vi "ADIS16460_Loop.vi"(8 "error in":errorcluster, 11 "ADI IMU Interrupt DevRef":T1={"ADI IMU DevRef"={"DevStatus"={"status"=FALSE, "code"=0, "source"=""}, "Handle"=0, "SPI Bus"=enum."SPI On-Board, CS0", "Device Found"=FALSE, "Device Ready"=FALSE, "Yaw Axis"=enum."Z", "AHRS Algorithm"=enum."Complementary"}, "InterruptRef"={"DevStatus"={"status"=FALSE, "code"=0, "source"=""}, "InterruptIndex"=enum."0"}}) -> (0 "error out":errorcluster, 1 "Device Found":bool)   [LabVIEW 2015, in "FRC ADIS16460.lvlib"]
doc: "Periodically reads the ADI MXP IMU valuse and makes data available for use elsewhere in your robot project. Place this block within PeriodicTasks.vi outside any loops."
uses:
  FRC ADIS16460.lvlib
  WPI_ADIS16460_InterruptDevRef.ctl
  WPI_ADIS16460_DevRef.ctl
  <vilib>/Rock Robotics/SystemInterfaces/spilib/spi_bus.ctl
  <vilib>/Rock Robotics/WPI/Interrupt/WPI_InterruptRef.ctl
  <vilib>/Rock Robotics/SystemInterfaces/Interrupt/FPGA_InterruptIndex.ctl
  <vilib>/Rock Robotics/WPI/SPI/WPI_SPIDevRef.ctl
  <vilib>/Platform/TimedLoop/XDataNode/timing_clust.ctl
  <vilib>/Platform/TimedLoop/XDataNode/nitl_modes.ctl
  <vilib>/Platform/TimedLoop/XDataNode/wakeup.ctl
  <vilib>/Analysis/baseanly.llb/Mean (DBL).vi
  <vilib>/Rock Robotics/SystemInterfaces/Interrupt/FPGA_WaitOnInterrupt.vi
  <vilib>/Rock Robotics/WPI/Utilities/WPI_UtilitiesTimebaseConstants.vi
  <vilib>/Rock Robotics/SystemInterfaces/Interrupt/FPGA_InterruptReadTimestamp.vi
  <vilib>/platform/TimedLoop/XDataNode/XDataNode.xnode
  <vilib>/Platform/TimedLoop/XDataNode/XDNodeRunTimeDep.lvlib
  <vilib>/Analysis/NI_AALBase.lvlib
panel:
  out "Loop Verification":i32
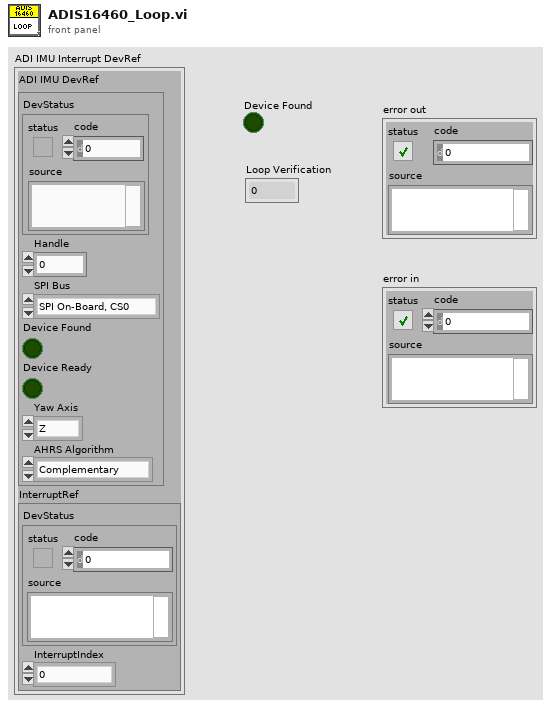
[diagram p1: front panel]
types:
  T1 = typedef "FRC ADIS16460.lvlib/WPI_ADIS16460_InterruptDevRef.ctl" = cluster{"ADI IMU DevRef":T2, "InterruptRef":T4}
  T2 = typedef "FRC ADIS16460.lvlib/WPI_ADIS16460_DevRef.ctl" = cluster{"DevStatus":errorcluster, "Handle":i32, "SPI Bus":T3, "Device Found":bool, "Device Ready":bool, "Yaw Axis":enum16{"X", "Y", "Z"}, "AHRS Algorithm":enum16{"Complementary", "Madgwick"}}
  T3 = typedef "spi_bus.ctl" = enum16{"SPI On-Board, CS0", "SPI On-Board, CS1", "SPI On-Board, CS2", "SPI On-Board, CS3", "SPI MXP", "Invalid"}
  T4 = typedef "WPI_InterruptRef.ctl" = cluster{"DevStatus":errorcluster, "InterruptIndex":T5}
  T5 = typedef "FPGA_InterruptIndex.ctl" = enum8{"0", "1", "2", "3", "4", "5", "6", "7", "Invalid"}
  T6 = typedef "WPI_SPIDevRef.ctl" = cluster{"DevStatus":errorcluster, "Handle":i32, "SPI Bus":T3}
  T7 = typedef "XDNodeRunTimeDep.lvlib/timing_clust.ctl" = cluster{"Expected End [f-1]":u64, "Actual End [f-1]":u64, "Finished Late? [f-1]":bool, "Expected End [i-1]":u64, "Actual End [i-1]":u64, "Finished Late? [i-1]":bool, "Expected Start [i]":u64, "Actual Start [i]":u64, "Expected Start [f]":u64, "Actual Start [f]":u64, "Source Name":string, "Structure Name":string, "Period":i64, "Deadline":i64, "Offset":i64, "Start":i64, "Priority":i32, "Timeout":i32, "Mode":T8, "Wakeup Reason":T9, "Error":errorcluster, "Source Type":string, "Secondary Source Type":string, "Global End Time":u64, "Global Start Time":u64, "Frame Duration":u64, "Iteration Duration":u64, "Assigned CPU":i32, "I/O Scan Engine Mode":u32}
  T8 = typedef "XDNodeRunTimeDep.lvlib/nitl_modes.ctl" = enum32{"No Change", "Process missed periods, maintain original phase", "Discard missed periods, maintain original phase", "Process missed periods, ignore original phase", "Discard missed periods, ignore original phase"}
  T9 = typedef "XDNodeRunTimeDep.lvlib/wakeup.ctl" = enum32{"Normal", "Aborted", "Asynchronous wakeup", "Timing source error", "Timed loop error", "Timeout"}
  T10 = cluster{"X Gyro Rate":dbl, "Y Gyro Rate":dbl, "Z Gyro Rate":dbl, "X Accel":dbl, "Y Accel":dbl, "Z Accel":dbl, "Temperature":dbl}
  T11 = cluster{"Output[0]":dbl, "Output[1]":dbl, "Output[2]":dbl}
  T12 = cluster{"Data Array[0]":dbl, "Data Array[1]":dbl, "Data Array[2]":dbl, "Data Array[3]":dbl, "Data Array[4]":dbl, "Data Array[5]":dbl, "Data Array[6]":dbl, "Data Array[7]":dbl, "Data Array[8]":dbl, "Data Array[9]":dbl, "Data Array[10]":dbl}
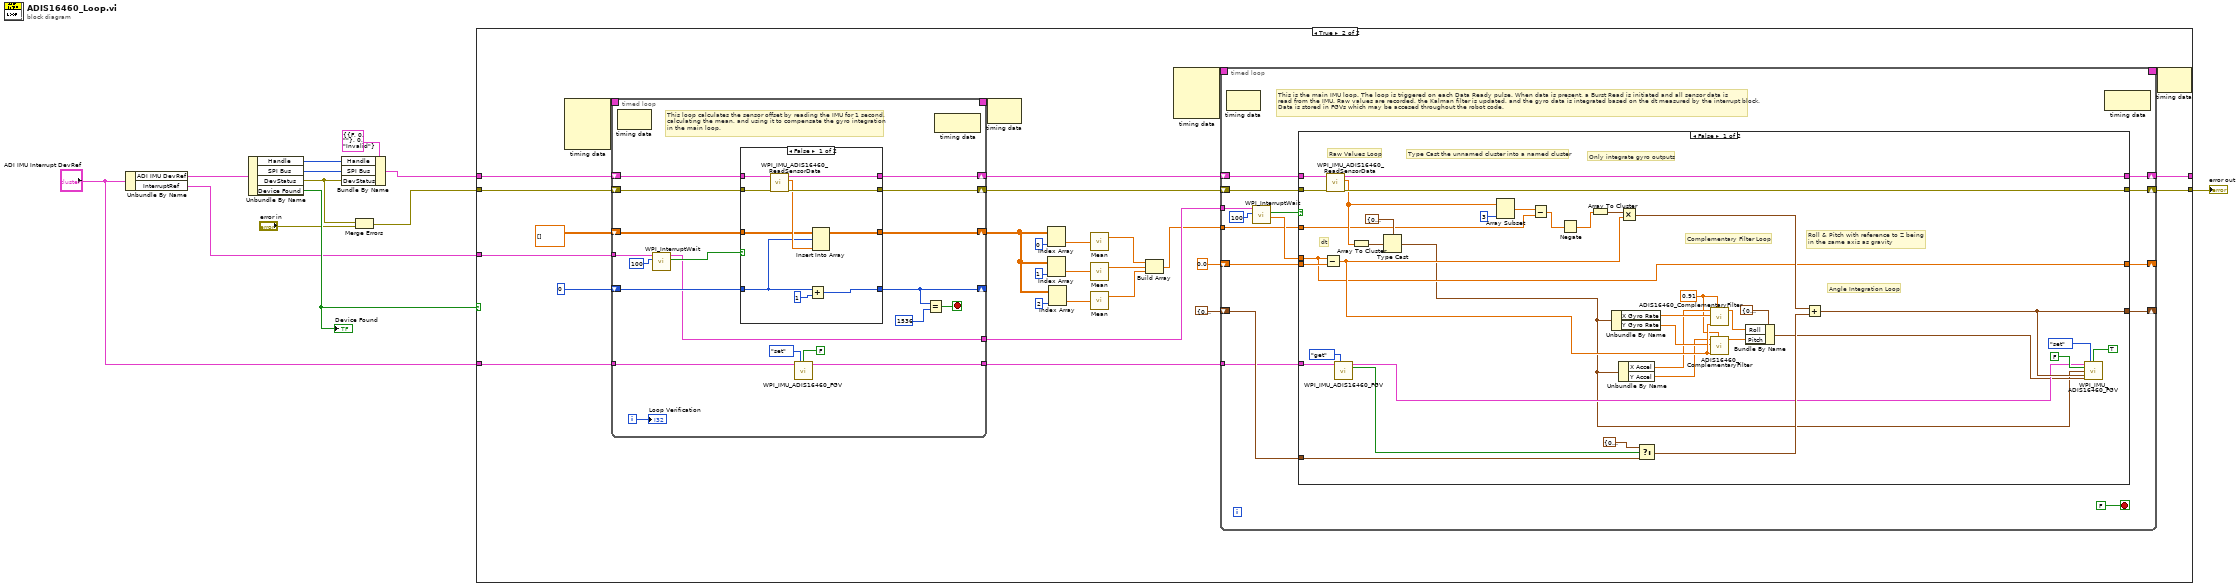
[diagram p0: block diagram]
diagram:
  n1 = Unbundle By Name("ADI IMU Interrupt DevRef") -> ("ADI IMU DevRef"=w6:T2, "InterruptRef"=w5:T4)
  n2 = Unbundle By Name(w6) -> ("Handle"=w11:i32, "SPI Bus"=w10:T3, "DevStatus"=w4:errorcluster, "Device Found"=w9:bool)
  "Device Found" <- w9
  n3 = Bundle By Name(cluster=T6 {"DevStatus"={"status"=FALSE, "code"=0, "source"=""}, "Handle"=0, "SPI Bus"=enum."Invalid"} ("SPIDevRef out"), "Handle"=w11, "SPI Bus"=w10, "DevStatus"=w4) -> (w8:T6)
  n4 = Merge Errors(w4, "error in") -> (w2:errorcluster)
  n5 = case shown="True" w9 {
    tunnel: w8 -> [w14 w23]
    tunnel: w2 -> [w13 w22]
    tunnel: [w13 w43] -> w7
    tunnel: [w14 w42] -> _
    tunnel: "ADI IMU Interrupt DevRef" -> [_ w18]
    tunnel: w5 -> [_ w19]
    frame False {
    }
    frame True {
      n6 = node-c288() -> (w37:T7)  [unwired: 4 in]
      n7 = timed-loop {
        shift-right: [w61] -> w21
        shift-left: w23 -> [w55]
        shift-right: [w62] -> w20
        shift-left: w22 -> [w54]
        shift-right: [w45] -> _
        shift-left: 0 -> [w59]
        tunnel: w19 -> [w58]
        tunnel: [w53] -> w16
        timing: w37 -> [_]
        timing-out: [_] -> w36
        tunnel: w18 -> [w51]
        tunnel: [w52] -> w17
        shift-right: [w60] -> w30
        shift-left: dbl[][] [] -> [w47]
        i -> [w48]
        stop <- w44 stop-if-true
        # "This loop calculates the sensor offset by reading the IMU for 1 second, \ncalculating the mean, and using it to compensate the gyro integration\nin the main loop."
        n8 = node-c288() -> ()  [unwired: 1 in, 1 out]
        n9 = call <vilib>:"WPI_InterruptWait.vi"("Timeout (ms)"=100, "InterruptRef"=w58) -> ("Timed Out"=w56:bool, "InterruptRef"=w53:T4)  [unwired: 5 in, 3 out]
        n10 = case shown="False" w56 {
          tunnel: [w74 w76] -> w62
          tunnel: [w73 w77] -> w61
          tunnel: [w65 w75] -> w60
          tunnel: w54 -> [w72 w76]
          tunnel: w55 -> [w71 w77]
          tunnel: w59 -> [w66 w78]
          tunnel: [w70 w78] -> w45
          tunnel: w47 -> [w67 w75]
          frame False {
            n11 = call "WPI_IMU_ADIS16460_ReadSensorData.vi"("error in (no error)"=w72, "SPIDevRef in"=w71) -> ("error out"=w74:errorcluster, "Data Array"=w68:dbl[], "SPIDevRef out"=w73:T6)  [unwired: 7 in]
            n12 = Add(x=w66, y=1) -> (x+y=w70:i32)
            n13 = Insert Into Array(array=w67, index (row)=w66, new element=w68) -> (w65:dbl[][])  [unwired: 1 in]
          }
          frame True {
          }
        }
        n14 = call "WPI_IMU_ADIS16460_FGV.vi"("ADI IMU Interrupt DevRef"=w51, "Operation"=enum16{"set", "get"}."set", "Sensor Ready?"=FALSE) -> ("ADI IMU Interrupt DevRef"=w52:T1)  [unwired: 7 in, 5 out]
        n15 = Equal?(x=w45, y=1536) -> (x = y?=w44:bool)
        n16 = node-c288() -> ()  [unwired: 1 in, 1 out]
        "Loop Verification" <- w48
      }
      n17 = node-c288(w36) -> ()  [unwired: 1 out]
      n18 = Index Array(array=w30, index (col)=0 ("disabled index (col)")) -> (element=w29:dbl[])  [unwired: 1 in]
      n19 = Index Array(array=w30, index (col)=1 ("disabled index (col)")) -> (element=w28:dbl[])  [unwired: 1 in]
      n20 = Index Array(array=w30, index (col)=2 ("disabled index (col)")) -> (element=w27:dbl[])  [unwired: 1 in]
      n21 = call-poly <vilib>:"Mean.vi"("X"=w29) -> ("mean"=w26:dbl)  [unwired: 1 out]
      n22 = call-poly <vilib>:"Mean.vi"("X"=w28) -> ("mean"=w25:dbl)  [unwired: 1 out]
      n23 = call-poly <vilib>:"Mean.vi"("X"=w27) -> ("mean"=w24:dbl)  [unwired: 1 out]
      n24 = Build Array(w26, w25, w24) -> (w15:dbl[])
      n25 = node-c288() -> (w39:T7)  [unwired: 4 in]
      n26 = timed-loop {
        shift-right: [w95] -> w42
        shift-left: w21 -> [w90]
        shift-right: [w94] -> w43
        shift-left: w20 -> [w89]
        shift-right: [w92] -> _
        shift-left: cluster{dbl, dbl, dbl} {0.0, 0.0, 0.0} -> [w91]
        tunnel: w16 -> [w87]
        shift-right: [w82] -> _
        shift-left: 0.0 ("TimeStamp") -> [w85]
        tunnel: w17 -> [w83]
        timing: w39 -> [_]
        timing-out: [_] -> w38
        tunnel: w15 -> [w81]
        stop <- FALSE stop-if-true
        # "This is the main IMU loop. The loop is triggered on each Data Ready pulse. When data is present, a Burst Read is initiated and all sensor data is \nread from the IMU. Raw values are recorded, the Kalman filter is updated, and the gyro data is integrated based on the dt measured by the interrupt block.\nData is stored in FGVs which may be accesed throughout the robot code."
        n27 = node-c288() -> ()  [unwired: 1 in, 1 out]
        n28 = call <vilib>:"WPI_InterruptWait.vi"("Timeout (ms)"=100, "InterruptRef"=w87) -> ("TimeStamp"=w86:dbl, "Timed Out"=w84:bool)  [unwired: 5 in, 3 out]
        n29 = case shown="False" w84 {
          tunnel: w90 -> [w135 w139]
          tunnel: w89 -> [w134 w138]
          tunnel: [w133 w139] -> w95
          tunnel: [w132 w138] -> w94
          tunnel: w83 -> [w122 _]
          tunnel: [w118 w137] -> w92
          tunnel: w91 -> [w128 w137]
          tunnel: w86 -> [w119 _]
          tunnel: w85 -> [w124 w136]
          tunnel: [w119 w136] -> w82
          tunnel: w81 -> [w100 _]
          frame False {
            w108 = 0.91
            # "Only integrate gyro outputs"
            # "Roll & Pitch with reference to Z being \nin the same axis as gravity"
            # "Type Cast the unnamed cluster into a named cluster"
            # "dt"
            # "Angle Integration Loop"
            # "Complementary Filter Loop"
            # "Raw Values Loop"
            n30 = Subtract(x=w119, y=w124) -> (x-y=w120:dbl)
            n31 = call "WPI_IMU_ADIS16460_ReadSensorData.vi"("error in (no error)"=w134, "SPIDevRef in"=w135) -> ("error out"=w132:errorcluster, "Data Array"=w113:dbl[], "SPIDevRef out"=w133:T6)  [unwired: 7 in]
            n32 = call "WPI_IMU_ADIS16460_FGV.vi"("ADI IMU Interrupt DevRef"=w122, "Operation"=enum16{"set", "get"}."get") -> ("ADI IMU Interrupt DevRef"=w115:T1, "Reset Out"=w116:bool)  [unwired: 8 in, 4 out]
            n33 = Array To Cluster(array=w113) -> (cluster=w103:T12)
            n34 = Type Cast(type=T10 {"X Gyro Rate"=0.0, "Y Gyro Rate"=0.0, "Z Gyro Rate"=0.0, "X Accel"=0.0, "Y Accel"=0.0, "Z Accel"=0.0, "Temperature"=0.0} ("IMU Data"), x=w103) -> (*(type *) &x=w102:T10)
            n35 = Array Subset(array=w113, length=3) -> (w101:dbl[])  [unwired: 1 in]
            n36 = Subtract(x=w101, y=w100) -> (x-y=w99:dbl[])
            n37 = Negate(x=w99) -> (-x=w98:dbl[])
            n38 = Array To Cluster(array=w98) -> (cluster=w126:cluster{"[0]":dbl, "[1]":dbl, "[2]":dbl})
            n39 = Unbundle By Name(w102) -> ("X Gyro Rate"=w112:dbl, "Y Gyro Rate"=w111:dbl)
            n40 = Unbundle By Name(w102) -> ("X Accel"=w110:dbl, "Y Accel"=w109:dbl)
            n41 = Multiply(x=w126, y=w120) -> (x*y=w125:cluster{"[0]":dbl, "[1]":dbl, "[2]":dbl})
            n42 = Select(t=T11 {"Output[0]"=0.0, "Output[1]"=0.0, "Output[2]"=0.0} ("cluster"), s=w116, f=w128) -> (s? t:f=w117:T11)
            n43 = call "ADIS16460_ComplementaryFilter.vi"("Filter Coefficient a"=w108, "dt (ms)"=w120, "Gyro (degrees/second)"=w112, "Accelerometer (degrees)"=w110) -> ("Filtered"=w107:dbl)  [unwired: 6 in, 1 out]
            n44 = call "ADIS16460_ComplementaryFilter.vi"("Filter Coefficient a"=w108, "dt (ms)"=w120, "Gyro (degrees/second)"=w111, "Accelerometer (degrees)"=w109) -> ("Filtered"=w106:dbl)  [unwired: 6 in, 1 out]
            n45 = Bundle By Name(cluster=cluster{"Pitch":dbl, "Roll":dbl} {"Pitch"=0.0, "Roll"=0.0} ("IMU AHRS OUT"), "Roll"=w107, "Pitch"=w106) -> (w114:cluster{"Pitch":dbl, "Roll":dbl})
            n46 = Add(x=w125, y=w117) -> (x+y=w118:cluster{dbl, dbl, dbl})
            n47 = call "WPI_IMU_ADIS16460_FGV.vi"("ADI IMU Interrupt DevRef"=w115, "Operation"=enum16{"set", "get"}."set", "Sensor Ready?"=TRUE, "Reset"=FALSE ("Calibrated"), "IMU Data"=w102, "IMU Angles"=w118, "IMU AHRS"=w114) -> ()  [unwired: 3 in, 6 out]
          }
          frame True {
            # "Waiting for an interrupt..."
          }
        }
        n48 = node-c288() -> ()  [unwired: 1 in, 1 out]
      }
      n49 = node-c288(w38) -> ()  [unwired: 1 out]
    }
  }
  "error out" <- w7
